vi "Memory.Pointer.Read Subset In Place (unsafe).vi"(7 "length":i64=-1 format="%d bytes", 8 "error in (no error)":errorcluster, 9 "offset (0)":u64 format="%d bytes", 10 "data in":string, 11 "Pointer in":refnum<class "Memory.Pointer.lvclass">) -> (0 "error out":errorcluster, 1 "offset dup":u64 format="%d bytes", 2 "data out":string, 3 "Pointer out":refnum<class "Memory.Pointer.lvclass">)   [LabVIEW 2016, in "LabVIEW Memory Manager.lvlib" / "Memory.Pointer.lvclass"]
uses:
  Memory.Pointer.lvclass
  Memory.Pointer.lvclass/Memory.Pointer.ctl
  Accessors/Memory.Pointer.Get Address.vi
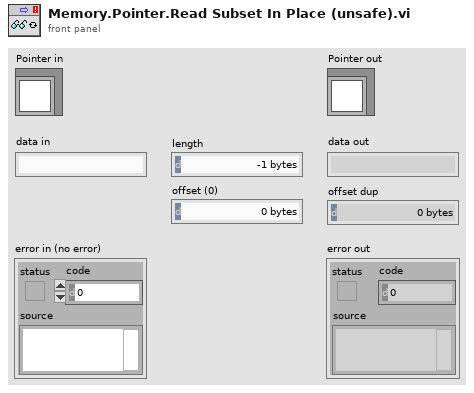
[diagram p1: front panel]
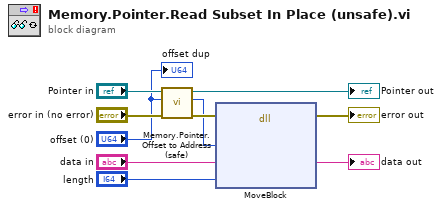
[diagram p0: block diagram]
diagram:
  n1 = call "Memory.Pointer.Offset to Address (safe).vi"("error in (no error)"="error in (no error)", "offset"="offset (0)", "Pointer in"="Pointer in") -> ("error out"=w10:errorcluster, "address"=w9:u64, "Pointer out"=→"Pointer out":refnum<class "Memory.Pointer.lvclass">)  [unwired: 5 in, 1 out]
  n2 = dll-call lib="LabVIEW" fn="MoveBlock"(error in=w10, "src pointer"=w9, "dst pointer"="data in", "size"="length") -> (error out=→"error out":errorcluster, "dst pointer"=→"data out":string)  [unwired: 5 in, 1 out]
  "offset dup" <- "offset (0)"
